vi "BIO_read.vi"(8 "error in (no error)":errorcluster, 9 "Timeout (10000ms)":u32=10000, 10 "bytes to read":i32=1024, 11 "BIO in":refnum<class "BIO.lvclass">) -> (0 "error out":errorcluster, 2 "Bytes read":u8[](array[numeric]), 3 "BIO out":refnum<class "BIO.lvclass">)   [LabVIEW 2013, in "SSL_Lib.lvlib" / "BIO.lvclass"]
uses:
  BIO.lvclass
  SSL-Lib/SSL-Lib.lvclass
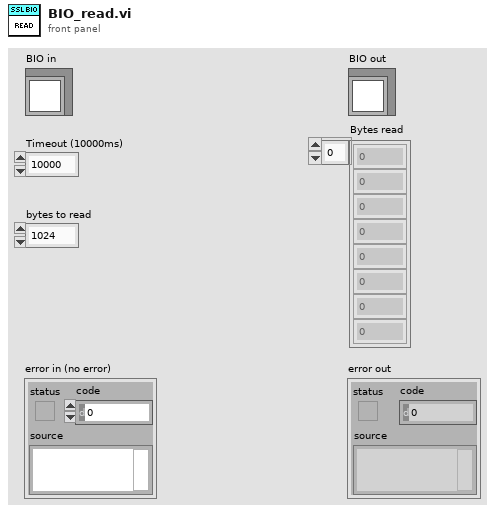
[diagram p1: front panel]
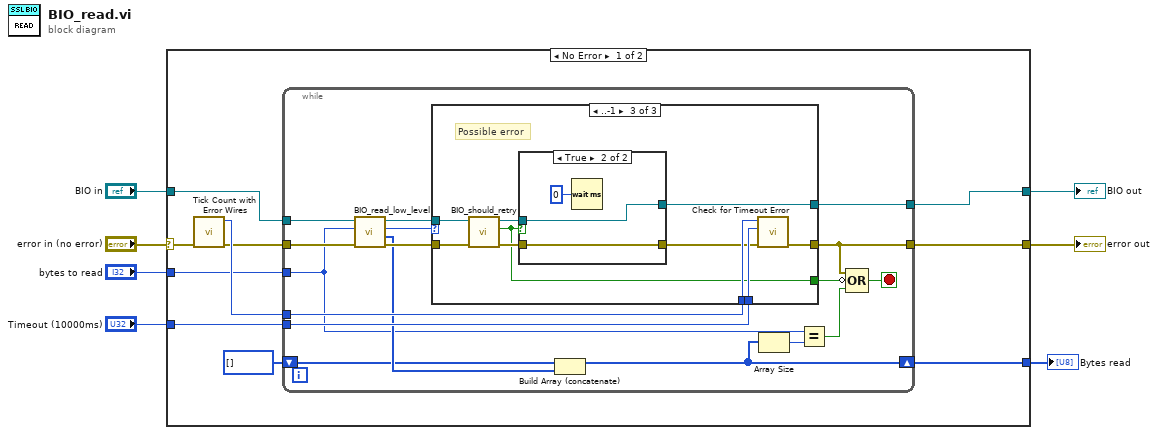
[diagram p0: block diagram]
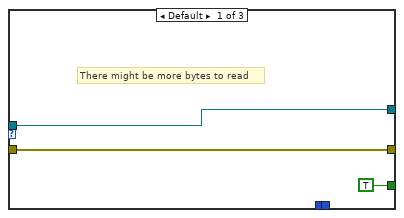
[diagram p2: hidden frame]
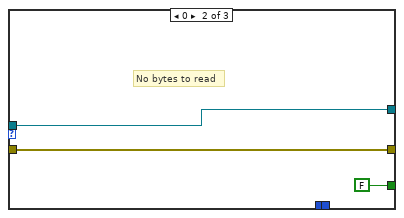
[diagram p3: hidden frame]
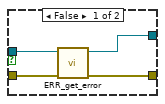
[diagram p4: hidden frame]
diagram:
  n1 = case shown="No Error" "error in (no error)" {
    selector: "error in (no error)" -> [w15 w59]
    tunnel: [w17 w59] -> w6
    tunnel: [w14 w58] -> w4
    tunnel: "BIO in" -> [w10 w58]
    tunnel: [w16 _] -> w3
    tunnel: "Timeout (10000ms)" -> [w12 _]
    tunnel: "bytes to read" -> [w9 _]
    frame No Error {
      n2 = call "Tick Count with Error Wires.vi"("error in (no error)"=w15) -> ("error out"=w11:errorcluster, "millisecond timer value"=w13:u32)  [unwired: 9 in]
      n3 = while {
        tunnel: w11 -> [w34]
        tunnel: [w31] -> w17
        tunnel: w10 -> [w24]
        tunnel: [w30] -> w14
        tunnel: w13 -> [w28]
        tunnel: w12 -> [w27]
        tunnel: w9 -> [w21]
        shift-right: [w18] -> w16
        shift-left: u8[] [] ("buf") -> [w19]
        stop <- w33 stop-if-true
        n4 = call "BIO_read_low_level.vi"("error in (no error)"=w34, "bytes to read"=w21, "BIO in"=w24) -> ("error out"=w32:errorcluster, "buf"=w23:u8[], "return type"=w26:i32, "BIO out"=w25:refnum<class "BIO.lvclass">)  [unwired: 5 in]
        n5 = case shown="..-1" w26 {
          tunnel: w32 -> [w36 w40 w50]
          tunnel: [w36 w40 w43] -> w31
          tunnel: w25 -> [w37 w39 w49]
          tunnel: [w37 w39 w46] -> w30
          tunnel: [TRUE ("Should retry") FALSE w41] -> w29
          tunnel: w28 -> [_ _ w44]
          tunnel: w27 -> [_ _ w45]
          frame Default {
            # "There might be more bytes to read"
          }
          frame 0 {
            # "No bytes to read"
          }
          frame ..-1 {
            # "Possible error"
            n6 = call "BIO_should_retry.vi"("error in (no error)"=w50, "BIO in"=w49) -> ("error out"=w48:errorcluster, "Should retry"=w41:bool, "BIO out"=w47:refnum<class "BIO.lvclass">)  [unwired: 7 in]
            n7 = case shown="True" w41 {
              tunnel: w48 -> [w54 w56]
              tunnel: [w53 w56] -> w42
              tunnel: w47 -> [w52 w57]
              tunnel: [w51 w57] -> w46
              frame False {
                n8 = call "ERR_get_error.vi"("error in (no error)"=w54, "SSL-Lib in"=w52) -> ("error out"=w53:errorcluster, "SSL-Lib out"=w51:refnum<class "BIO.lvclass">)  [unwired: 8 in]
              }
              frame True {
                n9 = Wait (ms)(milliseconds to wait=u32 0) -> ()  [unwired: 1 out]
              }
            }
            n10 = call "Check for Timeout Error.vi"("error in (no error)"=w42, "Timeout (10000ms)"=w45, "t0"=w44) -> ("error out"=w43:errorcluster)  [unwired: 8 in]
          }
        }
        n11 = Build Array (concatenate)(w19, w23) -> (w18:u8[])
        n12 = Array Size(array=w18) -> (size(s)=w22:i32)
        n13 = Equal?(x=w21, y=w22) -> (x = y?=w20:bool)
        n14 = Compound Arithmetic op=OR(w31, invert w29, w20) -> (w33:bool)
      }
    }
    frame Error {
    }
  }
  "error out" <- w6
  "BIO out" <- w4
  "Bytes read" <- w3
